vi "Configure Measurement (Duty Cycle).vi"(7 "Duty Cycle Type (0: Negative Duty Cycle Measurement)":i32(ring) items=["Negative Duty Cycle Measurement", "Positive Duty Cycle Measurement"], 8 "error in (no error)":errorcluster, 9 "Signal Reference Level (50 Percent)":dbl=50.0, 10 "Channel (1: Channel 1)":i32(ring)=1 items=["Channel 1"=1, "Channel 2"=2], 11 "VISA resource name":refnum<visa-resource-name>) -> (0 "error out":errorcluster, 3 "VISA resource name out":refnum<visa-resource-name>)   [LabVIEW 2024, in "Agilent 532XX Series.lvlib"]
doc: "Sets all measurement parameters and trigger parameters to default values for negative duty cycle measurements.\n\n<B>Note:</B> This VI only applies to the Agilent 53220A/53230A."
uses:
  Agilent 532XX Series.lvlib
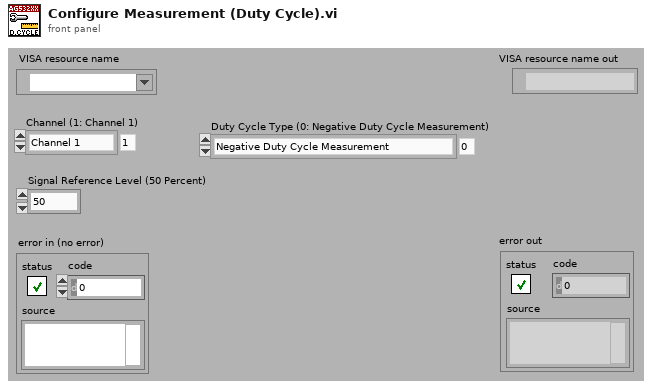
[diagram p1: front panel]
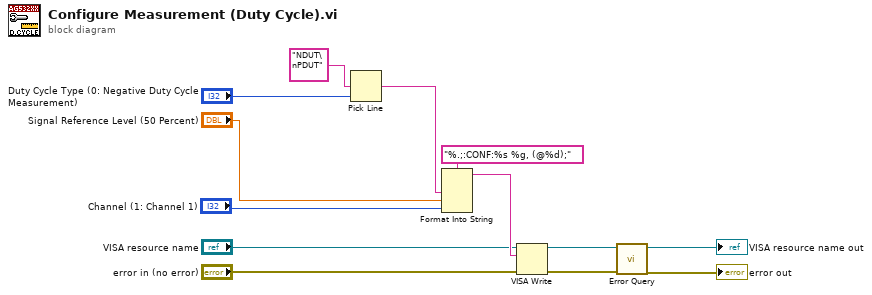
[diagram p0: block diagram]
diagram:
  n1 = Pick Line(multi-line string="NDUT\nPDUT", line index="Duty Cycle Type (0: Negative Duty Cycle Measurement)") -> (output string=w10:string)  [unwired: 1 out]
  n2 = Format Into String(format string="%.;:CONF:%s %g, (@%d);", w10, "Signal Reference Level (50 Percent)", "Channel (1: Channel 1)") -> (resulting string=w7:string)  [unwired: 2 in, 1 out]
  n3 = VISA Write(VISA resource name="VISA resource name", write buffer=w7, error in (no error)="error in (no error)") -> (VISA resource name out=w4:refnum<visa-resource-name>, error out=w3:errorcluster)  [unwired: 1 out]
  n4 = call "Error Query.vi"("error in (no error)"=w3, "VISA resource name"=w4) -> ("error out"=→"error out":errorcluster, "VISA resource name out"=→"VISA resource name out":refnum<visa-resource-name>)  [unwired: 8 out]
